vi "Nov_30 - Auto and Manual.vi"() -> ()   [LabVIEW 2020]
uses:
  <vilib>/Utility/error.llb/DialogType.ctl
  <vilib>/Analysis/3filter.llb/Filter Passband Type.ctl
  <vilib>/DAQmx/read.llb/DAQmx Read (Analog 1D DBL NChan 1Samp).vi
  <vilib>/DAQmx/create/channels.llb/DAQmx Create Channel (AI-Voltage-Basic).vi
  <vilib>/DAQmx/configure/timing.llb/DAQmx Timing (Sample Clock).vi
  <vilib>/DAQmx/miscellaneous.llb/DAQmx Fill In Error Info.vi
  <vilib>/Analysis/3filter.llb/Butterworth Filter (DBL).vi
  <vilib>/Utility/file.llb/Write Delimited Spreadsheet (string).vi
  <vilib>/Utility/file.llb/Write Delimited Spreadsheet (DBL).vi
  <vilib>/Analysis/NI_AALBase.lvlib
panel:
  out "Release":bool
  out "Pull":bool
  in  "Working Mode":string(combo)
  out "Load Cell":dbl
  in  "Pull CMD":bool
  in  "Release CMD":bool
  out "Load Cell":dynamicdata(graph)
  in  "Motor Trottle":dbl(slide) scale=0.0..5.0
  out "Swing (Consumer Loop)":bool
  in  "Master Stop":bool
  out "Consumer Loop Speed":u32
  out "Producer Loop Speed":u32
  out "Swing":bool
  out "Force Plate":dynamicdata(graph)
  out "Accelerometers":dynamicdata(graph)
  out "Enlapsed Time (sec)":dbl
  # "Motor Control"
  # "Indicators"
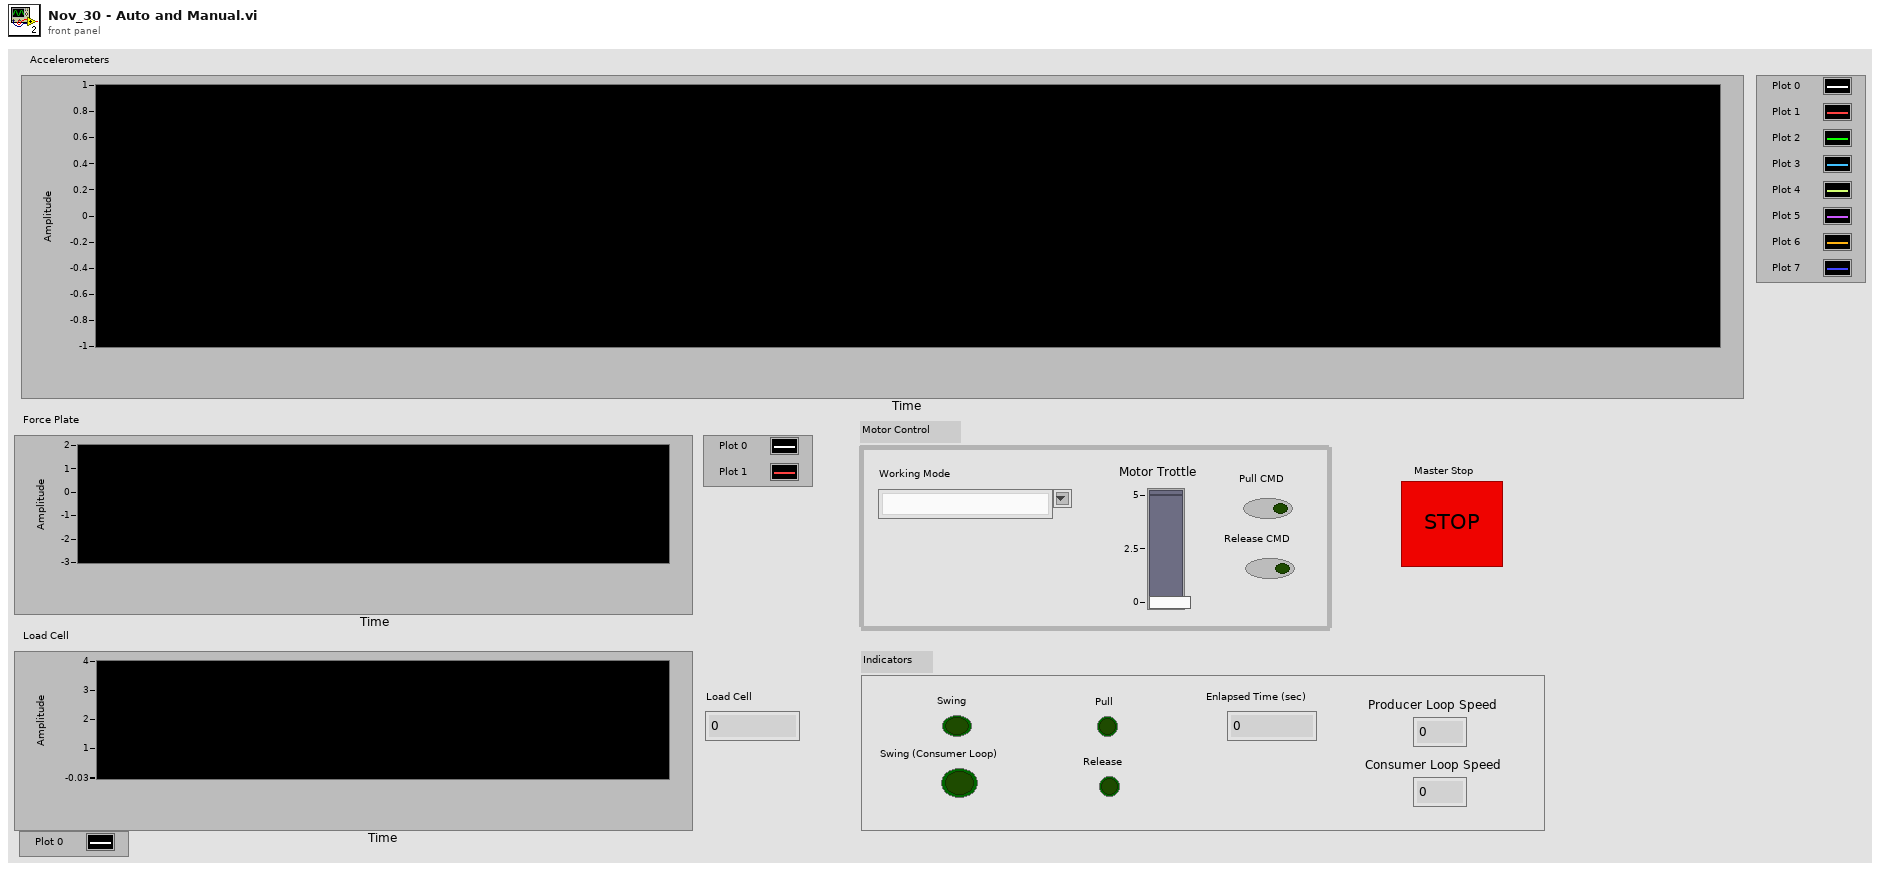
[diagram p1: front panel]
types:
  T1 = typedef "DialogType.ctl" = u16
  T2 = typedef "NI_AALBase.lvlib/Filter Passband Type.ctl" = enum32{"Lowpass", "Highpass", "Bandpass", "Bandstop"}
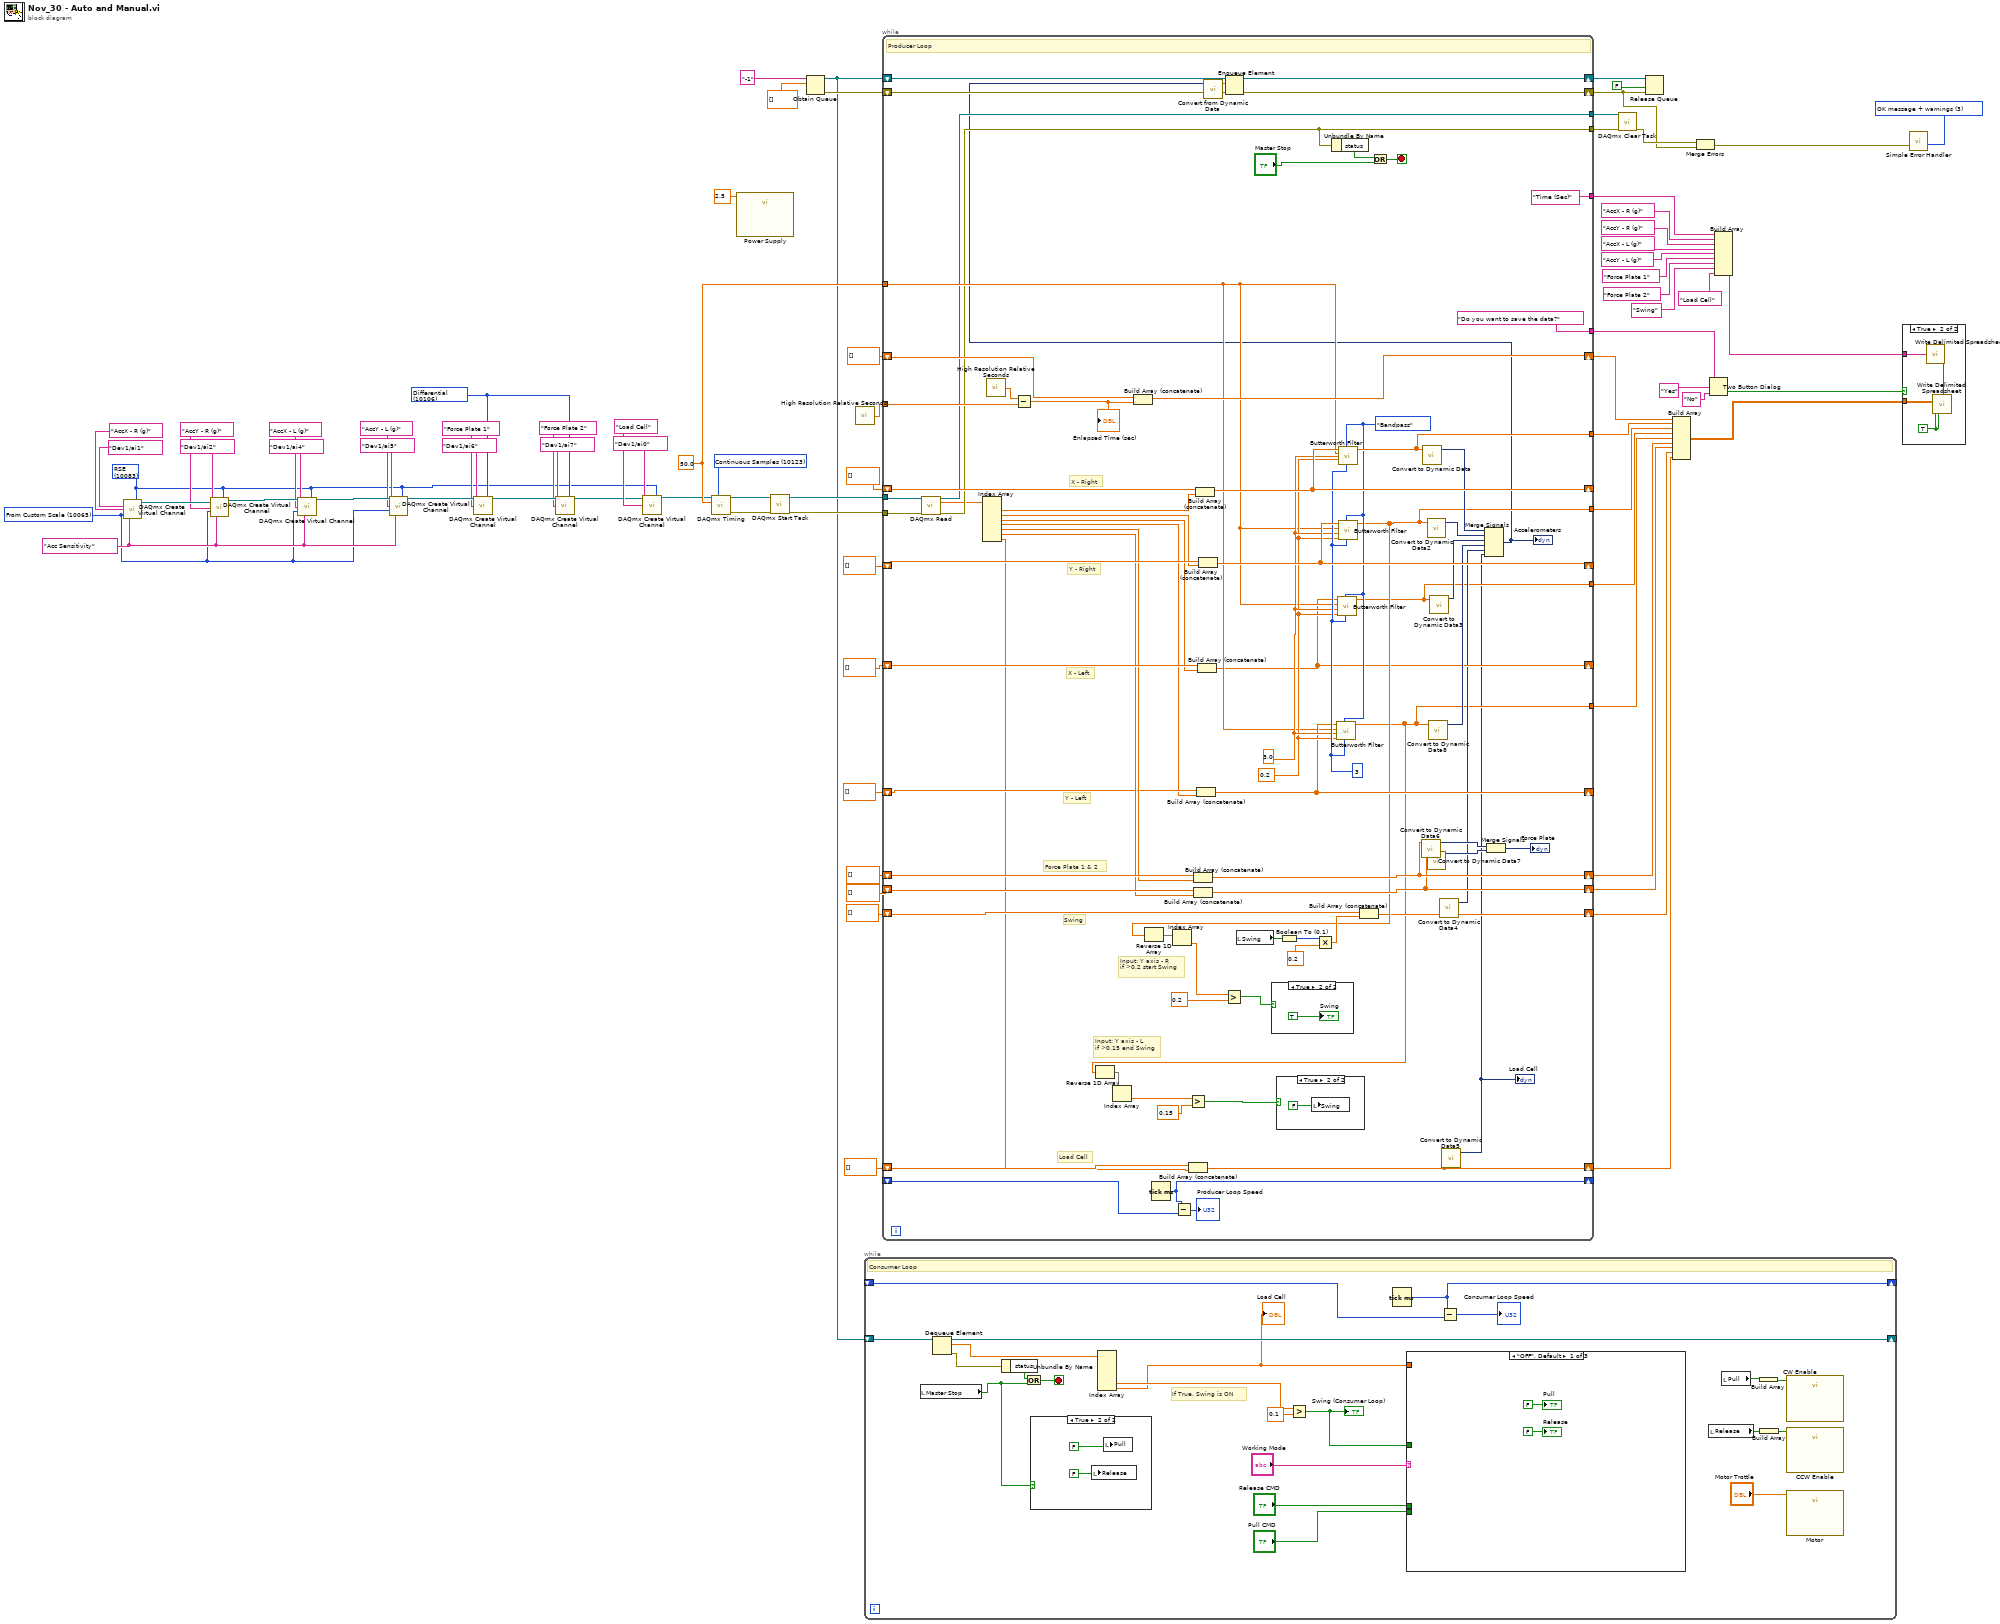
[diagram p0: block diagram]
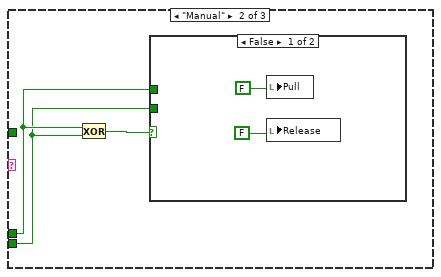
[diagram p3: hidden frame]
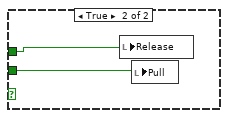
[diagram p4: hidden frame]
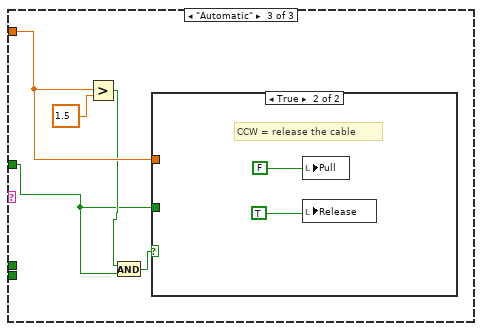
[diagram p5: hidden frame]
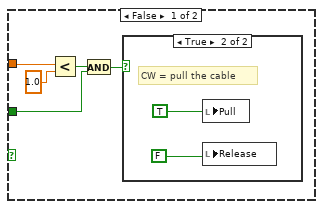
[diagram p6: hidden frame]
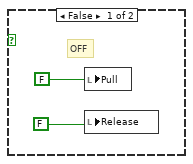
[diagram p7: hidden frame]
diagram:
  w15 = T1 3 items=["no dialog", "OK message", "continue or stop message", "OK message + warnings", "continue/stop + warnings"] ("type of dialog (OK msg:1)")
  w4 = 10065 items=["Volts"=10348, "From Custom Scale"=10065] ("units")
  w5 = tag "Acc Sensitivity" ("custom scale name")
  w25 = 10106 items=["Default"=-1, "RSE"=10083, "NRSE"=10078, "Differential"=10106, "Pseudodifferential"=12529] ("input terminal configuration")
  w47 = 10123 items=["Finite Samples"=10178, "Continuous Samples"=10123, "Hardware Timed Single Point"=12522] ("sample mode")
  w42 = 50.0 ("rate")
  w8 = 10083 items=["Default"=-1, "RSE"=10083, "NRSE"=10078, "Differential"=10106, "Pseudodifferential"=12529] ("input terminal configuration")
  n1 = call-poly <vilib>:"DAQmx Create Virtual Channel.vi"("input terminal configuration"=w8, "physical channels"=tag "Dev1/ai1" ("Physical channels"), "name to assign"="AccX - R (g)", "units"=w4, "custom scale name"=w5) -> ("task out"=w41:refnum<k21>)  [unwired: 9 in, 1 out]
  n2 = call-poly <vilib>:"DAQmx Create Virtual Channel.vi"("task in"=w41, "input terminal configuration"=w8, "physical channels"=tag "Dev1/ai2", "name to assign"="AccY - R (g)", "units"=w4, "custom scale name"=w5) -> ("task out"=w40:refnum<k21>)  [unwired: 8 in, 1 out]
  n3 = call-poly <vilib>:"DAQmx Create Virtual Channel.vi"("task in"=w40, "input terminal configuration"=w8, "physical channels"=tag "Dev1/ai4", "name to assign"="AccX - L (g)", "units"=w4, "custom scale name"=w5) -> ("task out"=w39:refnum<k21>)  [unwired: 8 in, 1 out]
  n4 = call-poly <vilib>:"DAQmx Create Virtual Channel.vi"("task in"=w39, "input terminal configuration"=w8, "physical channels"=tag "Dev1/ai5", "name to assign"="AccY - L (g)", "units"=w4, "custom scale name"=w5) -> ("task out"=w38:refnum<k21>)  [unwired: 8 in, 1 out]
  n5 = call-poly <vilib>:"DAQmx Create Virtual Channel.vi"("task in"=w38, "input terminal configuration"=w25, "physical channels"=tag "Dev1/ai6", "name to assign"="Force Plate 1" ("element")) -> ("task out"=w32:refnum<k21>)  [unwired: 10 in, 1 out]
  n6 = call-poly <vilib>:"DAQmx Create Virtual Channel.vi"("task in"=w32, "input terminal configuration"=w25, "physical channels"=tag "Dev1/ai7", "name to assign"="Force Plate 2" ("element")) -> ("task out"=w7:refnum<k21>)  [unwired: 10 in, 1 out]
  n7 = call-poly <vilib>:"DAQmx Create Virtual Channel.vi"("task in"=w7, "input terminal configuration"=w8, "physical channels"=tag "Dev1/ai0", "name to assign"="Load Cell") -> ("task out"=w6:refnum<k21>)  [unwired: 10 in, 1 out]
  n8 = call-poly <vilib>:"DAQmx Timing.vi"("task/channels in"=w6, "sample mode"=w47, "rate"=w42) -> ("task out"=w46:refnum<k21>, "error out"=w45:errorcluster)  [unwired: 11 in]
  n9 = call "Power Supply"("data"=2.5) -> ()  [unwired: 17 in, 2 out]
  n10 = call <vilib>:"DAQmx Start Task.vi"("task/channels in"=w46, "error in"=w45) -> ("task out"=w44:refnum<k21>, "error out"=w43:errorcluster)  [unwired: 12 in]
  n11 = Obtain Queue(name (unnamed)="-1", element data type=dbl[] []) -> (queue out=w11:refnum<queue>, error out=w20:errorcluster)  [unwired: 3 in, 1 out]
  n12 = call <vilib>:"High Resolution Relative Seconds.vi"() -> ("relative seconds"=w78:dbl)
  n13 = while {
    shift-right: [w99] -> _
    shift-left: w11 -> [w100]
    shift-right: [w96] -> _
    shift-left: _ -> [w97]
    stop <- w94 stop-if-true
    # "If True, Swing is ON"
    # "Consumer Loop"
    n14 = local read "Master Stop"() -> (w79:bool)
    n15 = Dequeue Element(queue=w100) -> (queue out=w99:refnum<queue>, element=w92:dbl[], error out=w93:errorcluster)  [unwired: 2 in, 1 out]
    n16 = Unbundle By Name(w93) -> ("status"=w95:bool)
    n17 = Or(x=w95, y=w79) -> (x .or. y?=w94:bool)
    n18 = case shown="True" w79 {
      frame False {
      }
      frame True {
        n19 = local write "Release"(FALSE) -> ()
        n20 = local write "Pull"(FALSE) -> ()
      }
    }
    n21 = Index Array(array=w92) -> (element #5=w91:dbl, element #6=w89:dbl)  [unwired: 6 in, 4 out]
    "Load Cell" <- w89
    n22 = Greater?(x=w91, y=0.1) -> (0:w80:bool)
    "Swing (Consumer Loop)" <- w80
    n23 = Tick Count (ms)() -> (millisecond timer value=w96:u32)
    n24 = case shown="\"OFF\", Default" "Working Mode" {
      tunnel: w89 -> [_ _ w115]
      tunnel: "Release CMD" -> [_ w106 _]
      tunnel: "Pull CMD" -> [_ w105 _]
      tunnel: w80 -> [_ _ w112]
      frame "OFF", Default {
        "Pull" <- FALSE
        "Release" <- FALSE
      }
      frame "Manual" {
        n25 = Exclusive Or(1:w105, 2:w106) -> (0:w107:bool)
        n26 = case shown="False" w107 {
          tunnel: w106 -> [_ w110]
          tunnel: w105 -> [_ w111]
          frame False {
            n27 = local write "Pull"(FALSE) -> ()
            n28 = local write "Release"(FALSE) -> ()
          }
          frame True {
            n29 = local write "Release"(w110) -> ()
            n30 = local write "Pull"(w111) -> ()
          }
        }
      }
      frame "Automatic" {
        n31 = Greater?(x=w115, y=1.5) -> (0:w113:bool)
        n32 = And(x=w113, y=w112) -> (x .and. y?=w114:bool)
        n33 = case shown="True" w114 {
          tunnel: w115 -> [w121 _]
          tunnel: w112 -> [w117 _]
          frame False {
            n34 = Less?(x=w121, y=1.0) -> (x < y?=w118:bool)
            n35 = And(x=w118, y=w117) -> (x .and. y?=w119:bool)
            n36 = case shown="True" w119 {
              frame False {
                # "OFF"
                n37 = local write "Pull"(FALSE) -> ()
                n38 = local write "Release"(FALSE) -> ()
              }
              frame True {
                # "CW = pull the cable"
                n39 = local write "Pull"(TRUE) -> ()
                n40 = local write "Release"(FALSE) -> ()
              }
            }
          }
          frame True {
            # "CCW = release the cable"
            n41 = local write "Pull"(FALSE) -> ()
            n42 = local write "Release"(TRUE) -> ()
          }
        }
      }
    }
    n43 = Subtract(x=w96, y=w97) -> (x-y=→"Consumer Loop Speed":u32)
    n44 = local read "Release"() -> (w83:bool)
    n45 = local read "Pull"() -> (w84:bool)
    n46 = Build Array(w84) -> (w86:bool[])
    n47 = Build Array(w83) -> (w85:bool[])
    n48 = call "Motor"("data"="Motor Trottle") -> ()  [unwired: 17 in, 2 out]
    n49 = call "CW Enable"("data"=w86) -> ()  [unwired: 17 in, 2 out]
    n50 = call "CCW Enable"("data"=w85) -> ()  [unwired: 17 in, 2 out]
  }
  n51 = while {
    tunnel: w44 -> [w204]
    tunnel: w43 -> [w203]
    tunnel: w78 -> [w201]
    shift-right: [w185] -> w75
    shift-left: dbl[] [] -> [w199]
    shift-right: [w189] -> _
    shift-left: dbl[] [] -> [w198]
    shift-right: [w188] -> _
    shift-left: dbl[] [] -> [w197]
    tunnel: ["Time (Sec)"] -> w50
    tunnel: ["Do you want to save the data?" ("message")] -> w67
    shift-right: [w149] -> w54
    shift-left: dbl[] [] -> [w194]
    shift-right: [w150] -> _
    shift-left: dbl[] [] -> [w186]
    shift-right: [w175] -> w52
    shift-left: dbl[] [] -> [w178]
    shift-right: [w173] -> w53
    shift-left: dbl[] [] -> [w177]
    tunnel: [w171] -> w57
    tunnel: [w153] -> w56
    tunnel: [w145] -> w55
    shift-right: [w164] -> _
    shift-left: dbl[] [] -> [w163]
    tunnel: [w144] -> w51
    tunnel: w42 -> [w161]
    shift-right: [w155] -> _
    shift-left: _ -> [w154]
    shift-right: [w138] -> w19
    shift-left: w11 -> [w139]
    shift-right: [w136] -> w12
    shift-left: w20 -> [w137]
    tunnel: [w143] -> w17
    tunnel: [w140] -> w16
    shift-right: [w131] -> w2
    shift-left: dbl[] [] -> [w130]
    stop <- w141 stop-if-true
    w168 = 3 ("order")
    w166 = 0.2 ("low cutoff freq: fl")
    w167 = 3.0 ("high cutoff freq: fh")
    w162 = Filter_Passband_Type."Bandpass" ("filter type")
    # "X - Right"
    # "Y - Right"
    # "X - Left"
    # "Y - Left"
    # "Force Plate 1 & 2"
    # "Swing"
    # "Load Cell"
    # "Input: Y axis - L\nif >0.15 end Swing"
    # "Input: Y axis - R\nif >0.2 start Swing"
    # "Producer Loop"
    n52 = call-poly <vilib>:"DAQmx Read.vi"("task/channels in"=w204, "error in"=w203) -> ("task out"=w143:refnum<k21>, "data"=w135:dbl[], "error out"=w140:errorcluster)  [unwired: 11 in]
    n53 = Index Array(array=w135) -> (element #1=w160:dbl, element #2=w159:dbl, element #3=w158:dbl, element #4=w157:dbl, element #5=w169:dbl, element #6=w170:dbl, element #7=w129:dbl)  [unwired: 7 in]
    n54 = call <vilib>:"High Resolution Relative Seconds.vi"() -> ("relative seconds"=w202:dbl)
    n55 = Subtract(x=w202, y=w201) -> (x-y=w200:dbl)
    "Enlapsed Time (sec)" <- w200
    n56 = Build Array (concatenate)(w199, w200) -> (w185:dbl[])
    n57 = Tick Count (ms)() -> (millisecond timer value=w155:u32)
    n58 = Subtract(x=w155, y=w154) -> (x-y=→"Producer Loop Speed":u32)
    n59 = Build Array (concatenate)(w130, w129) -> (w131:dbl[])
    n60 = Build Array (concatenate)(w178, w169) -> (w175:dbl[])
    n61 = Build Array (concatenate)(w177, w170) -> (w173:dbl[])
    n62 = Build Array (concatenate)(w198, w160) -> (w189:dbl[])
    n63 = Build Array (concatenate)(w163, w157) -> (w164:dbl[])
    n64 = Build Array (concatenate)(w186, w158) -> (w150:dbl[])
    n65 = Build Array (concatenate)(w197, w159) -> (w188:dbl[])
    n66 = local read "Swing"() -> (w187:bool)
    n67 = Boolean To (0,1)(Boolean=w187) -> (0, 1=w192:i16)
    n68 = Multiply(x=w192, y=0.2) -> (x*y=w193:dbl)
    n69 = Unbundle By Name(w140) -> ("status"=w142:bool)
    n70 = call-poly <vilib>:"Butterworth Filter.vi"("order"=w168, "filter type"=w162, "low cutoff freq: fl"=w166, "high cutoff freq: fh"=w167, "sampling freq: fs"=w161, "X"=w164) -> ("Filtered X"=w144:dbl[])  [unwired: 2 in, 1 out]
    n71 = Reverse 1D Array(array=w144) -> (reversed array=w180:dbl[])
    n72 = Index Array(array=w180) -> (element=w179:dbl)  [unwired: 1 in]
    n73 = Greater?(x=w179, y=0.15) -> (0:w147:bool)
    n74 = case shown="True" w147 {
      frame False {
      }
      frame True {
        n75 = local write "Swing"(FALSE) -> ()
      }
    }
    n76 = call-poly <vilib>:"Butterworth Filter.vi"("order"=w168, "filter type"=w162, "low cutoff freq: fl"=w166, "high cutoff freq: fh"=w167, "sampling freq: fs"=w161, "X"=w150) -> ("Filtered X"=w145:dbl[])  [unwired: 2 in, 1 out]
    n77 = call-poly <vilib>:"Butterworth Filter.vi"("order"=w168, "filter type"=w162, "low cutoff freq: fl"=w166, "high cutoff freq: fh"=w167, "sampling freq: fs"=w161, "X"=w189) -> ("Filtered X"=w171:dbl[])  [unwired: 2 in, 1 out]
    n78 = call-poly <vilib>:"Butterworth Filter.vi"("order"=w168, "filter type"=w162, "low cutoff freq: fl"=w166, "high cutoff freq: fh"=w167, "sampling freq: fs"=w161, "X"=w188) -> ("Filtered X"=w153:dbl[])  [unwired: 2 in, 1 out]
    n79 = Reverse 1D Array(array=w153) -> (reversed array=w190:dbl[])
    n80 = Index Array(array=w190) -> (element=w152:dbl)  [unwired: 1 in]
    n81 = Greater?(x=w152, y=0.2) -> (0:w146:bool)
    n82 = case shown="True" w146 {
      frame False {
      }
      frame True {
        "Swing" <- TRUE
      }
    }
    n83 = Build Array (concatenate)(w194, w193) -> (w149:dbl[])
    n84 = Or(x=w142, y="Master Stop") -> (x .or. y?=w141:bool)
    n85 = call "Convert to Dynamic Data6"("Array"=w175) -> ("Dynamic Data Type"=w174:dynamicdata)  [unwired: 3 in]
    n86 = call "Convert to Dynamic Data"("Array"=w171) -> ("Dynamic Data Type"=w184:dynamicdata)  [unwired: 3 in]
    n87 = call "Convert to Dynamic Data2"("Array"=w153) -> ("Dynamic Data Type"=w183:dynamicdata)  [unwired: 3 in]
    n88 = call "Convert to Dynamic Data7"("Array"=w173) -> ("Dynamic Data Type"=w172:dynamicdata)  [unwired: 3 in]
    n89 = call "Convert to Dynamic Data8"("Array"=w144) -> ("Dynamic Data Type"=w165:dynamicdata)  [unwired: 3 in]
    n90 = call "Convert to Dynamic Data3"("Array"=w145) -> ("Dynamic Data Type"=w182:dynamicdata)  [unwired: 3 in]
    n91 = call "Convert to Dynamic Data4"("Array"=w149) -> ("Dynamic Data Type"=w148:dynamicdata)  [unwired: 3 in]
    n92 = call "Convert to Dynamic Data5"("Array"=w131) -> ("Dynamic Data Type"=w128:dynamicdata)  [unwired: 3 in]
    "Load Cell" <- w128
    n93 = Merge Signals(w184, w183, w182, w165, w148, w128) -> (w133:dynamicdata)
    "Accelerometers" <- w133
    n94 = call "Convert from Dynamic Data"("Dynamic Data Type"=w133) -> ("Array"=w132:dbl[])  [unwired: 3 in]
    n95 = Enqueue Element(queue=w139, element=w132, error in (no error)=w137) -> (queue out=w138:refnum<queue>, error out=w136:errorcluster)  [unwired: 1 in, 1 out]
    n96 = Merge Signals(w174, w172) -> (→"Force Plate":dynamicdata)
  }
  n97 = call <vilib>:"DAQmx Clear Task.vi"("task in"=w17, "error in"=w16) -> ("error out"=w13:errorcluster)  [unwired: 13 out]
  n98 = Release Queue(queue=w19, force destroy? (F)=FALSE, error in (no error)=w12) -> ()  [unwired: 3 out]
  n99 = Build Array(w75, w57, w56, w55, w51, w52, w53, w54, w2) -> (w74:dbl[][])
  n100 = Merge Errors(w13, w12) -> (w14:errorcluster)
  n101 = Two Button Dialog(message=w67, 1:"No" ("F button name (\"Cancel\")"), 2:"Yes" ("T button name (\"OK\")")) -> (T button?=w70:bool)
  n102 = Build Array(w50, "AccX - R (g)", "AccY - R (g)", "AccX - L (g)", "AccY - L (g)", "Force Plate 1" ("element"), "Force Plate 2" ("element"), "Swing" ("element"), "Load Cell" ("element")) -> (w73:string[])
  n103 = case shown="True" w70 {
    tunnel: w74 -> [_ w210]
    tunnel: w73 -> [_ w209]
    frame False {
    }
    frame True {
      w208 = TRUE ("transpose? (no:F)")
      n104 = call-poly <vilib>:"Write Delimited Spreadsheet.vi"("1D data"=w209) -> ("new file path (Not A Path if cancelled)"=w207:path)  [unwired: 13 in, 1 out]
      n105 = call-poly <vilib>:"Write Delimited Spreadsheet.vi"("file path (dialog if empty)"=w207, "2D data"=w210, "append to file? (new file:F)"=w208, "transpose? (no:F)"=w208) -> ()  [unwired: 10 in, 2 out]
    }
  }
  n106 = call <vilib>:"Simple Error Handler.vi"("type of dialog (OK msg:1)"=w15, "error in (no error)"=w14) -> ()  [unwired: 8 out]
